vi "Read XY from Tag To ClusterArray.vi"(10 "Input TagArray":refnum<class "Tag.lvclass">[](array[class])) -> (2 "Tag ClusterArray Out":cluster{"TagID":dbl, "TagX":dbl, "TagY":dbl}[](array[cluster]))   [LabVIEW 2014]
doc: "This VI reads input Tag array and converts it to ArrayCluster with XY values per Tag object"
uses:
  Tag.lvclass
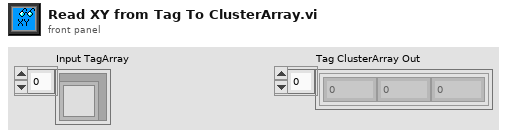
[diagram p1: front panel]
types:
  T1 = cluster{"TagID":dbl, "RealTagX":dbl, "RealTagY":dbl}
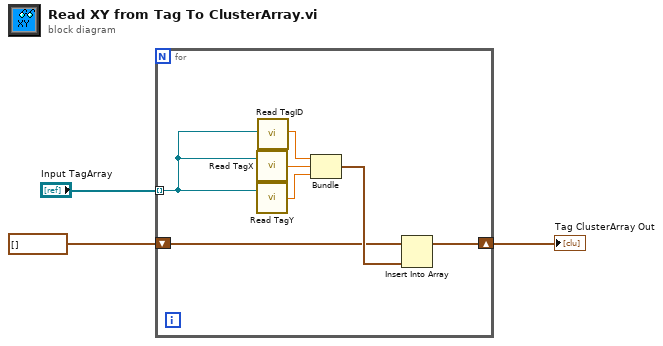
[diagram p0: block diagram]
diagram:
  n1 = for {
    tunnel: "Input TagArray" -> [w5] mode=indexing
    shift-right: [w6] -> w1
    shift-left: cluster{"TagID":dbl, "TagX":dbl, "TagY":dbl}[] [] ("Tag ClusterArray Out") -> [w7]
    n2 = call-dynamic "Read TagX.vi"("Tag in"=w5) -> ("RealTagX"=w10:dbl)  [unwired: 1 in, 2 out]
    n3 = call-dynamic "Read TagY.vi"("Tag in"=w5) -> ("RealTagY"=w9:dbl)  [unwired: 1 in, 2 out]
    n4 = call "Read TagID.vi"("Tag in"=w5) -> ("TagID"=w4:dbl)  [unwired: 16 in, 2 out]
    n5 = Bundle("TagID"=w4, "RealTagX"=w10, "RealTagY"=w9) -> (w8:T1)  [unwired: 1 in]
    n6 = Insert Into Array(array=w7, new element=w8) -> (w6:cluster{"TagID":dbl, "TagX":dbl, "TagY":dbl}[])  [unwired: 1 in]
  }
  "Tag ClusterArray Out" <- w1
